vi "Process.vi"(8 "error in (no error)":errorcluster, 10 "pound in":refnum<class "Pound.lvclass">, 11 "qbus in":refnum<class "Qbus.lvclass">) -> (0 "error out":errorcluster)   [LabVIEW 2015, in "FileHandler.lvlib"]
doc: "Implements timer tasks that other processes register by sending Qbus messages to those processes."
uses:
  FileHandler.lvlib
  <vilib>/addons/Qbus/Qbus.lvclass
  <vilib>/NI/Software Watchdog/Pound/Pound.lvclass
  controls/ProcessState.ctl
  <vilib>/drjdpowell/SQLite Library/SQL Connection/Connection.lvclass
  <vilib>/NI/Software Watchdog/Watchdog/Watchdog.lvclass
  CopyUtility/CopyUtility.lvlib
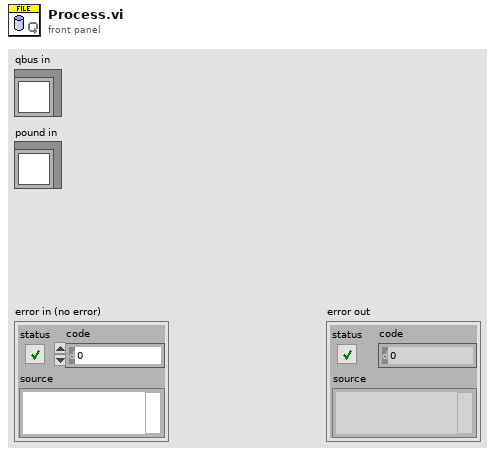
[diagram p1: front panel]
types:
  T1 = typedef "FileHandler.lvlib/ProcessState.ctl" = cluster{"SQLite Connection":refnum<class "Connection.lvclass">}
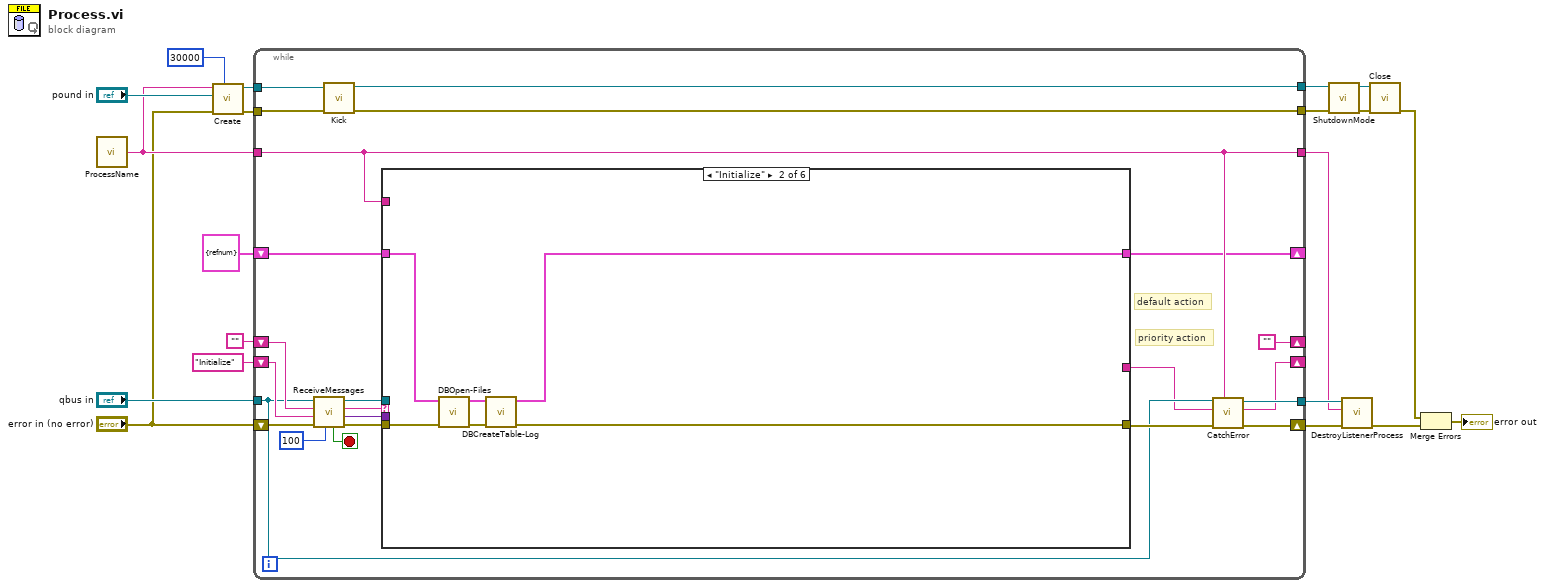
[diagram p0: block diagram]
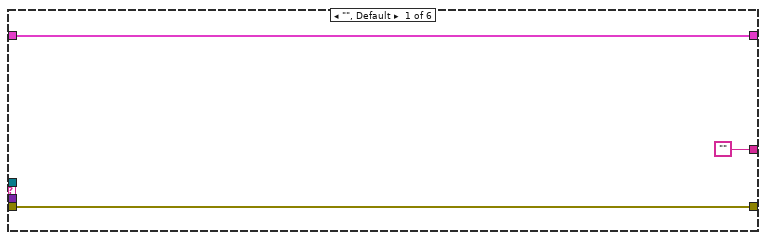
[diagram p2: hidden frame]
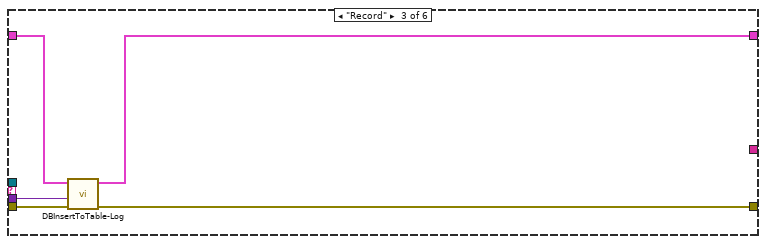
[diagram p3: hidden frame]
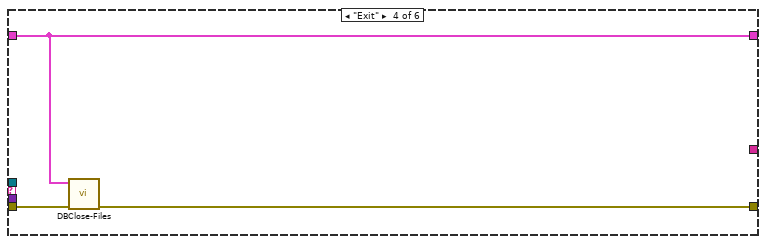
[diagram p4: hidden frame]
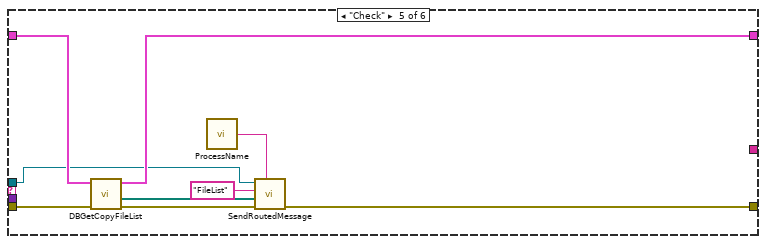
[diagram p5: hidden frame]
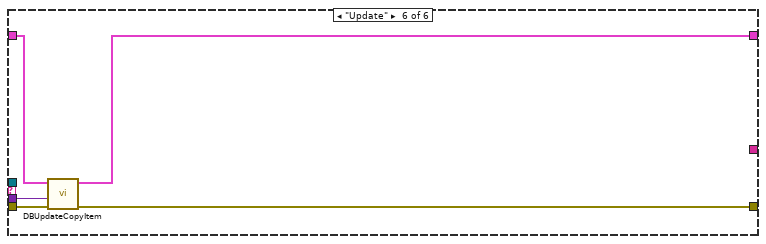
[diagram p6: hidden frame]
diagram:
  n1 = call "ProcessName.vi"() -> ("process name"=w11:string)  [unwired: 5 in]
  n2 = call <vilib>:"Create.vi"("Execution Timeout (ms)"=u32 30000, "error in (no error)"="error in (no error)", "Pound"="pound in", "Name"=w11) -> ("error out"=w13:errorcluster, "Watchdog"=w12:refnum<data-value>)  [unwired: 6 in]
  n3 = while {
    shift-right: [""] -> _
    shift-left: "" -> [w41]
    tunnel: "qbus in" -> [w25]
    tunnel: w11 -> [w32]
    tunnel: [w34] -> w18
    tunnel: [w32] -> w17
    shift-right: [w33] -> _
    shift-left: "Initialize" -> [w36]
    tunnel: w13 -> [w30]
    tunnel: w12 -> [w29]
    tunnel: [w28] -> w6
    tunnel: [w27] -> w7
    shift-right: [w35] -> w19
    shift-left: "error in (no error)" -> [w43]
    shift-right: [w22] -> _
    shift-left: T1 {"SQLite Connection"=refnum} ("ProcessState") -> [w23]
    stop <- w42 stop-if-true
    # "priority action"
    # "default action"
    n4 = call "ReceiveMessages.vi"("timeout(100)"=100, "error in (no error)"=w43, "priority action"=w36, "default action"=w41, "qbus in"=w25) -> ("error out"=w40:errorcluster, "message value"=w37:variant, "action"=w26:string, "qbus out"=w38:refnum<class "Qbus.lvclass">, "exit"=w42:bool)  [unwired: 2 in]
    n5 = call <vilib>:"Kick.vi"("error in (no error)"=w30, "Watchdog"=w29) -> ("error out"=w27:errorcluster, "Watchdog"=w28:refnum<data-value>)  [unwired: 8 in]
    n6 = case shown="\"Initialize\"" w26 {
      tunnel: w40 -> [w46 w52 w57 w60 w69 w74]
      tunnel: w38 -> [_ _ _ _ w63 _]
      tunnel: [w46 w47 w53 w58 w61 w70] -> w31
      tunnel: w37 -> [_ _ w56 _ _ w73]
      tunnel: w32 -> [_ _ _ _ _ _]
      tunnel: w23 -> [w45 w51 w55 w59 w68 w72]
      tunnel: [w45 w48 w54 w59 w67 w71] -> w22
      tunnel: ["" _ _ _ _ _] -> w21
      frame "", Default {
      }
      frame "Initialize" {
        n7 = call "DBOpen-Files.vi"("error in (no error)"=w52, "ProcessState in"=w51) -> ("error out"=w49:errorcluster, "ProcessState out"=w50:T1)  [unwired: 8 in]
        n8 = call "DBCreateTable-Log.vi"("error in (no error)"=w49, "ProcessState in"=w50) -> ("error out"=w47:errorcluster, "ProcessState out"=w48:T1)  [unwired: 8 in]
      }
      frame "Record" {
        n9 = call "DBInsertToTable-Log.vi"("error in (no error)"=w57, "message value"=w56, "ProcessState in"=w55) -> ("error out"=w53:errorcluster, "ProcessState out"=w54:T1)  [unwired: 7 in]
      }
      frame "Exit" {
        n10 = call "DBClose-Files.vi"("error in (no error)"=w60, "ProcessState in"=w59) -> ("error out"=w58:errorcluster)  [unwired: 9 in]
      }
      frame "Check" {
        n11 = call "DBGetCopyFileList.vi"("error in (no error)"=w69, "ProcessState in"=w68) -> ("error out"=w66:errorcluster, "FilePaths"=w65:path[], "ProcessState out"=w67:T1)  [unwired: 7 in]
        n12 = call "ProcessName.vi"() -> ("process name"=w62:string)  [unwired: 5 in]
        n13 = call <vilib>:"SendRoutedMessage.vi"("listener process"=w62, "error in (no error)"=w66, "message value"=w65, "message name"="FileList", "Qbus in"=w63) -> ("error in (no error)"=w61:errorcluster)  [unwired: 5 in, 1 out]
      }
      frame "Update" {
        n14 = call "DBUpdateCopyItem.vi"("error in (no error)"=w74, "message value"=w73, "ProcessState in"=w72) -> ("error out"=w70:errorcluster, "ProcessState out"=w71:T1)  [unwired: 7 in]
      }
    }
    n15 = call <vilib>:"CatchError.vi"("source"=w32, "error in (no error)"=w31, "next action in"=w21, "Qbus in"=w25) -> ("error out"=w35:errorcluster, "next action out"=w33:string, "Qbus out"=w34:refnum<class "Qbus.lvclass">)  [unwired: 5 in]
  }
  n16 = call <vilib>:"ShutdownMode.vi"("error in (no error)"=w7, "Watchdog"=w6) -> ("error out"=w8:errorcluster, "Watchdog"=w9:refnum<data-value>)  [unwired: 8 in]
  n17 = call <vilib>:"DestroyListenerProcess.vi"("error in (no error)"=w19, "process name"=w17, "Qbus in"=w18) -> ("error in (no error)"=w4:errorcluster)  [unwired: 7 in, 1 out]
  n18 = call <vilib>:"Close.vi"("error in (no error)"=w8, "Watchdog"=w9) -> ("error out"=w5:errorcluster)  [unwired: 9 in]
  n19 = Merge Errors(w5, w4) -> (→"error out":errorcluster)
